vi "Test SequencerV2.vi"(0 "TestRunning?":bool, 1 "WaitingData":bool, 2 "StepDataActive":dbl format="%#_13g", 3 "ProgramMode":T1, 4 "StepTimeLimit":dbl format="%#_13g", 5 "State Array In":string[](array[string]), 6 "Stabilized?":bool, 7 "LastDataTime":i64, 8 "GrabManual":bool, 9 "StableCount":dbl format="%#_13g", 10 "CmdHeld":dbl format="%#_13g") -> (14 "FreezeCmdPID":bool, 16 "Next Timed Point":dbl, 19 "State Array Out":string[](array[string]))   [LabVIEW 2013]
uses:
  TypeDef/ProgramMode(PC).ctl
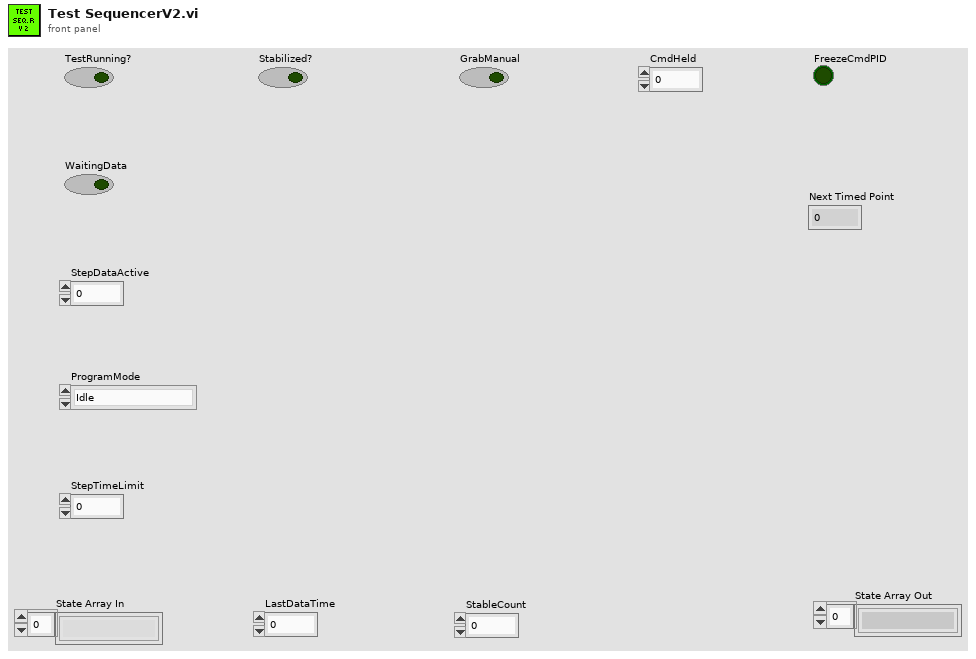
[diagram p1: front panel]
types:
  T1 = typedef "ProgramMode(PC).ctl" = enum16{"Idle", "Manual", "Flow", "Fix Data Point", "Guided Flow", "Timed Test", "Hot Fuel"}
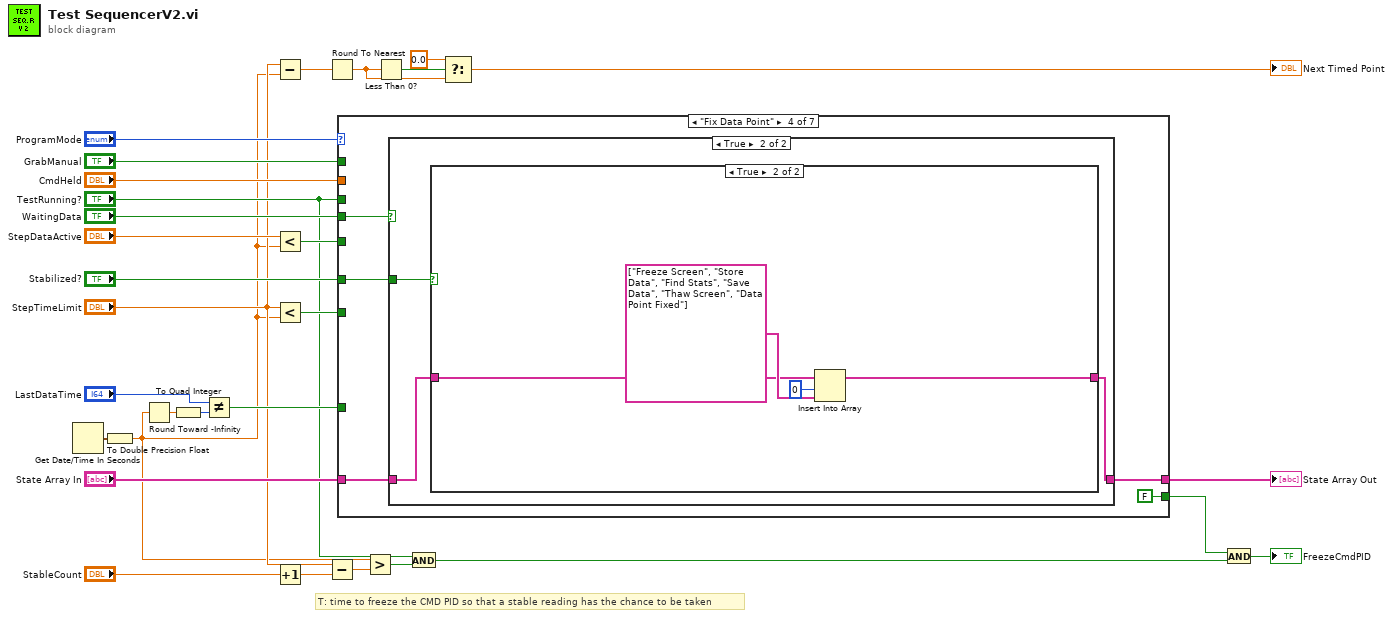
[diagram p0: block diagram]
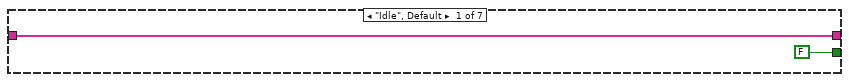
[diagram p2: hidden frame]
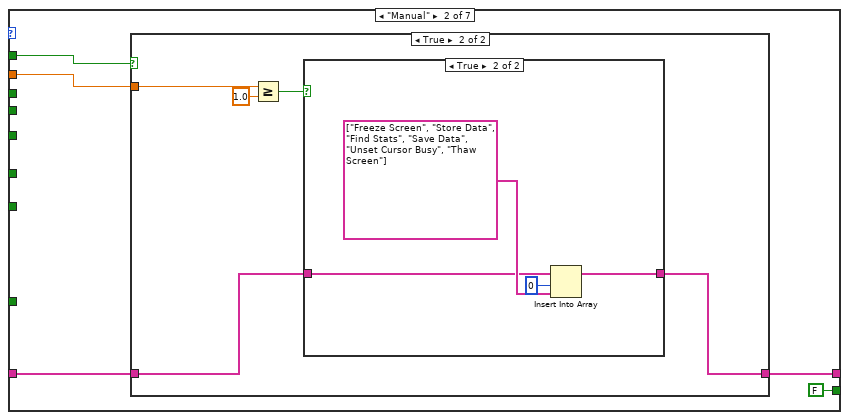
[diagram p3: hidden frame]
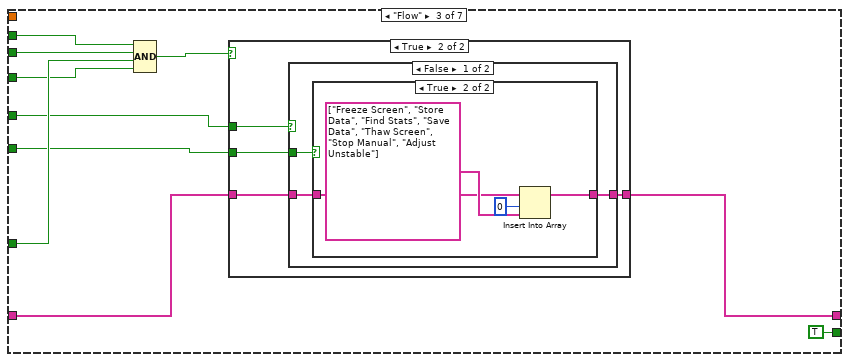
[diagram p6: hidden frame]
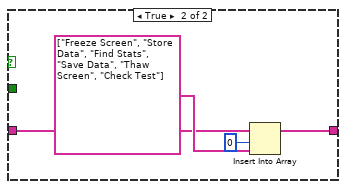
[diagram p9: hidden frame]
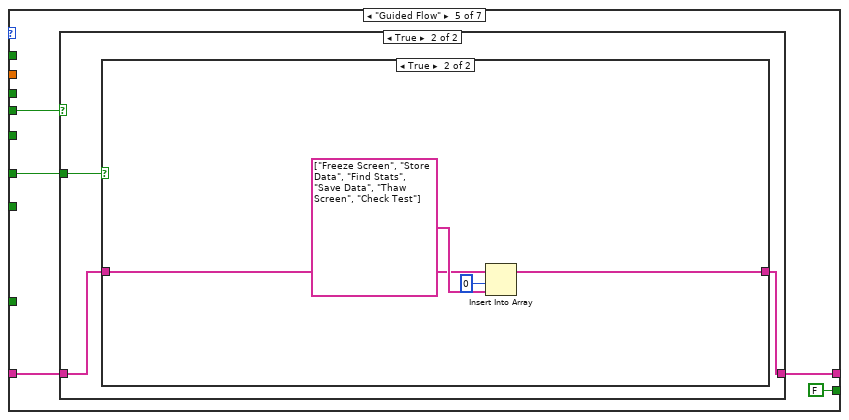
[diagram p12: hidden frame]
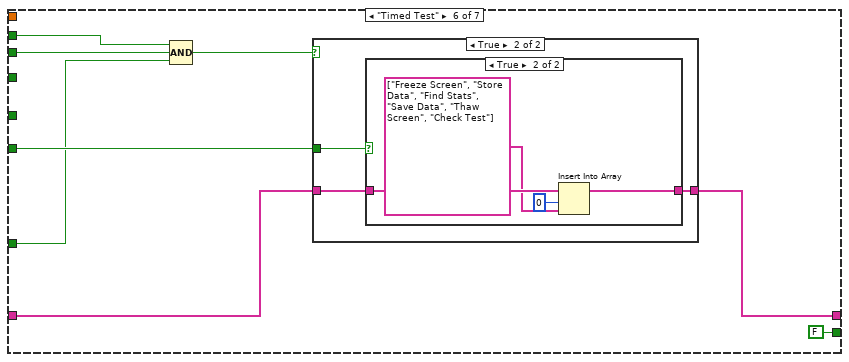
[diagram p15: hidden frame]
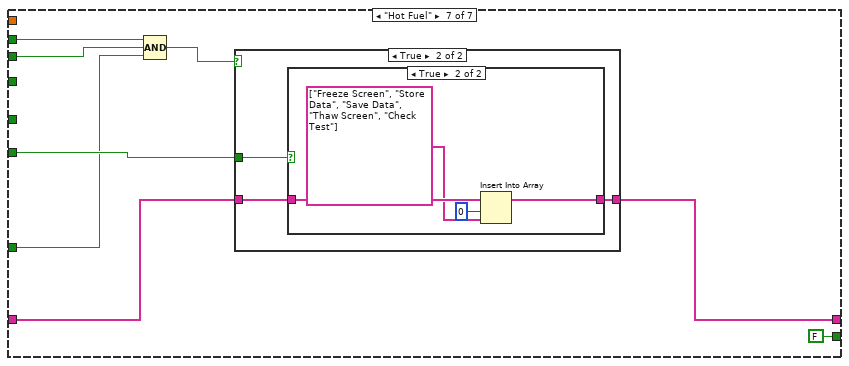
[diagram p18: hidden frame]
diagram:
  # "T: time to freeze the CMD PID so that a stable reading has the chance to be taken"
  n1 = Get Date/Time In Seconds() -> (seconds since 1Jan1904=w26:timestamp)
  n2 = To Double Precision Float(number=w26) -> (double precision float=w6:dbl)
  n3 = Round Toward -Infinity(1:w6) -> (0:w25:dbl)
  n4 = To Quad Integer(1:w25) -> (0:w27:i64)
  n5 = Not Equal?(x="LastDataTime", y=w27) -> (x != y?=w21:bool)
  n6 = Subtract(x="StepTimeLimit", y=w6) -> (x-y=w5:dbl)
  n7 = Less?(x="StepDataActive", y=w6) -> (x < y?=w19:bool)
  n8 = Less?(x="StepTimeLimit", y=w6) -> (x < y?=w23:bool)
  n9 = Increment(x="StableCount") -> (x+1=w15:dbl)
  n10 = Round To Nearest(number=w5) -> (nearest integer value=w3:dbl)
  n11 = Subtract(x="StepTimeLimit", y=w15) -> (x-y=w16:dbl)
  n12 = case shown="\"Fix Data Point\"" "ProgramMode" {
    tunnel: "State Array In" -> [w32 w36 w58 w80 w92 w111 w128]
    tunnel: [w32 w35 w57 w79 w91 w110 w127] -> w12
    tunnel: "GrabManual" -> [_ w37 _ _ _ _ _]
    tunnel: "CmdHeld" -> [_ w34 _ _ _ _ _]
    tunnel: w23 -> [_ _ w53 _ _ w109 w123]
    tunnel: "WaitingData" -> [_ _ w55 w78 w94 w106 w124]
    tunnel: "TestRunning?" -> [_ _ w56 _ _ w108 w125]
    tunnel: w21 -> [_ _ w54 _ _ w107 w122]
    tunnel: w19 -> [_ _ w52 _ _ _ _]
    tunnel: "Stabilized?" -> [_ _ w50 w77 w93 _ _]
    tunnel: [FALSE FALSE TRUE FALSE FALSE FALSE FALSE] -> w11
    frame "Idle", Default {
    }
    frame "Manual" {
      n13 = case shown="True" w37 {
        tunnel: w36 -> [w38 w40]
        tunnel: [w38 w39] -> w35
        tunnel: w34 -> [_ w42]
        frame False {
        }
        frame True {
          n14 = Greater Or Equal?(x=w42, y=1.0) -> (x >= y?=w41:bool)
          n15 = case shown="True" w41 {
            tunnel: w40 -> [w44 w45]
            tunnel: [w44 w46] -> w39
            frame False {
            }
            frame True {
              n16 = Insert Into Array(array=w45, index=0, new element=string[] ["Freeze Screen", "Store Data", "Find Stats", "Save Data", "Unset Cursor Busy", "Thaw Screen"]) -> (w46:string[])
            }
          }
        }
      }
    }
    frame "Flow" {
      n17 = Compound Arithmetic op=AND(w56, w55, w54, w52) -> (w51:bool)
      n18 = case shown="True" w51 {
        tunnel: w58 -> [w59 w63]
        tunnel: [w59 w62] -> w57
        tunnel: w53 -> [_ w61]
        tunnel: w50 -> [_ w60]
        frame False {
        }
        frame True {
          n19 = case shown="False" w60 {
            tunnel: w63 -> [w66 w73]
            tunnel: [w65 w72] -> w62
            tunnel: w61 -> [w64 _]
            frame False {
              n20 = case shown="True" w64 {
                tunnel: w66 -> [w67 w69]
                tunnel: [w67 w68] -> w65
                frame False {
                }
                frame True {
                  n21 = Insert Into Array(array=w69, index=0, new element=string[] ["Freeze Screen", "Store Data", "Find Stats", "Save Data", "Thaw Screen", "Stop Manual", "Adjust Unstable"]) -> (w68:string[])
                }
              }
            }
            frame True {
              n22 = Insert Into Array(array=w73, index=0, new element=string[] ["Freeze Screen", "Store Data", "Find Stats", "Save Data", "Thaw Screen", "Check Test"]) -> (w72:string[])
            }
          }
        }
      }
    }
    frame "Fix Data Point" {
      n23 = case shown="True" w78 {
        tunnel: w77 -> [_ w84]
        tunnel: w80 -> [w81 w83]
        tunnel: [w81 w82] -> w79
        frame False {
        }
        frame True {
          n24 = case shown="True" w84 {
            tunnel: w83 -> [w85 w87]
            tunnel: [w85 w86] -> w82
            frame False {
            }
            frame True {
              n25 = Insert Into Array(array=w87, index=0, new element=string[] ["Freeze Screen", "Store Data", "Find Stats", "Save Data", "Thaw Screen", "Data Point Fixed"]) -> (w86:string[])
            }
          }
        }
      }
    }
    frame "Guided Flow" {
      n26 = case shown="True" w94 {
        tunnel: w93 -> [_ w98]
        tunnel: w92 -> [w95 w97]
        tunnel: [w95 w96] -> w91
        frame False {
        }
        frame True {
          n27 = case shown="True" w98 {
            tunnel: w97 -> [w99 w101]
            tunnel: [w99 w100] -> w96
            frame False {
            }
            frame True {
              n28 = Insert Into Array(array=w101, index=0, new element=string[] ["Freeze Screen", "Store Data", "Find Stats", "Save Data", "Thaw Screen", "Check Test"]) -> (w100:string[])
            }
          }
        }
      }
    }
    frame "Timed Test" {
      n29 = Compound Arithmetic op=AND(w108, w106, w107) -> (w105:bool)
      n30 = case shown="True" w105 {
        tunnel: w111 -> [w112 w115]
        tunnel: [w112 w114] -> w110
        tunnel: w109 -> [_ w113]
        frame False {
        }
        frame True {
          n31 = case shown="True" w113 {
            tunnel: w115 -> [w116 w119]
            tunnel: [w116 w117] -> w114
            frame False {
            }
            frame True {
              n32 = Insert Into Array(array=w119, index=0, new element=string[] ["Freeze Screen", "Store Data", "Find Stats", "Save Data", "Thaw Screen", "Check Test"]) -> (w117:string[])
            }
          }
        }
      }
    }
    frame "Hot Fuel" {
      n33 = Compound Arithmetic op=AND(w125, w124, w122) -> (w126:bool)
      n34 = case shown="True" w126 {
        tunnel: w128 -> [w129 w132]
        tunnel: [w129 w131] -> w127
        tunnel: w123 -> [_ w130]
        frame False {
        }
        frame True {
          n35 = case shown="True" w130 {
            tunnel: w132 -> [w133 w136]
            tunnel: [w133 w134] -> w131
            frame False {
            }
            frame True {
              n36 = Insert Into Array(array=w136, index=0, new element=string[] ["Freeze Screen", "Store Data", "Save Data", "Thaw Screen", "Check Test"]) -> (w134:string[])
            }
          }
        }
      }
    }
  }
  "State Array Out" <- w12
  n37 = Greater?(x=w6, y=w16) -> (0:w17:bool)
  n38 = Less Than 0?(x=w3) -> (x < 0?=w4:bool)
  n39 = And(x="TestRunning?", y=w17) -> (x .and. y?=w10:bool)
  n40 = Select(t=0.0, s=w4, f=w3) -> (s? t:f=→"Next Timed Point":dbl)
  n41 = And(x=w11, y=w10) -> (x .and. y?=→"FreezeCmdPID":bool)
